vi "Stop Segmented Log.vi"(8 "error in (no error)":errorcluster, 11 "Segmented Log in":refnum<class "Segmented Log.lvclass">) -> (0 "error out":errorcluster, 3 "Instance File Paths":path[](array[path]))   [LabVIEW 2012, in "Waveform Data Logger Engine.lvlib" / "Segmented Log.lvclass"]
doc: "Closes the current log file instance and returns the final list of instance file paths."
uses:
  Segmented Log.lvclass
  Segmented Log.lvclass/Segmented Log.ctl
  On Segmented Log Complete.vi
  On File Close.vi
  Log Files/Log File/Close Log File.vi
  Make File Read-Only.vi
  Log Files/Log File/Log File.lvclass
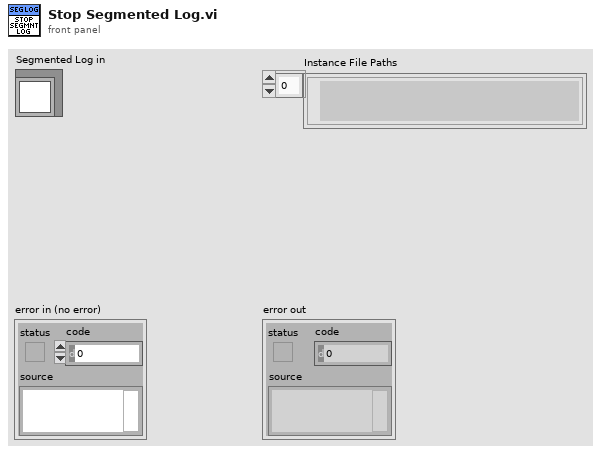
[diagram p1: front panel]
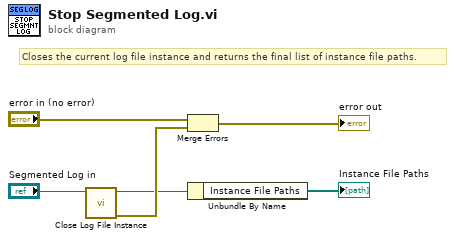
[diagram p0: block diagram]
diagram:
  # "Closes the current log file instance and returns the final list of instance file paths."
  n1 = call "Close Log File Instance.vi"("Segmented Log in"="Segmented Log in") -> ("error out"=w4:errorcluster, "Segmented Log out"=w2:refnum<class "Segmented Log.lvclass">)  [unwired: 9 in]
  n2 = Merge Errors("error in (no error)", w4) -> (→"error out":errorcluster)
  n3 = Unbundle By Name(w2) -> ("Instance File Paths"=→"Instance File Paths":path[])
